vi "AttackerNormal.vi"(4 "AI Parameters":T1={"GotoKick"={"Dist do cone a frente"=150.0, "attacker farback"=1500.0, "Perto"=300.0, "min dist to kick"=150.0, "kick eps"=0.05, "Time to transition"=0.0}, "Attacker"={"CC chute"=0.09, "CC passe"=0.045, "Kick Force"=100.0, "D ball-robot Kick"=200.0, "D ball-robot Pass"=0.3}, "Defender"={"D max"=1700.0, "Vel p/ robô av"=1000.0, "Kick Force"=100.0, "D atk-def"=0.0, "D farback"=0.0}, "Timeout"={"Field/v in x"=6.0, "Dist Robots"=300, "Dist up in y"=300}, "Pose Striker"={"dist"=200.0, "Numeric"=-4.0, "dist 2"=200.0}, "Dist Stop"=300.0, "Distance when ball out"=200, "D central gap "=150.0, "T pass"=0.0, "Force ++"=0.0, "range kick"=0.0, "Chute alto"=TRUE, "Marcador novo"=TRUE} {"D central gap" format="%#_13g"; "Dist Stop" format="%#_13g"; "Pose Striker"."Numeric" format="%#_13g"; "Defender"."Kick Force" format="%#_13g"; "Defender"."Vel p/ robô av" format="%#_13g"; "Attacker"."D ball-robot Kick" format="%#_13g"; "Attacker"."Kick Force" format="%#_13g"; "Attacker"."CC passe" format="%#_13g"; "Attacker"."CC chute" format="%#_13g"; "GotoKick"."kick eps" format="%#_13g"; "GotoKick"."min dist to kick" format="%#_13g"; "GotoKick"."Perto" format="%#_13g"; "GotoKick"."attacker farback" format="%#_13g"; "GotoKick"."Dist do cone a frente" format="%#_13g"}, 5 "Penalty":bool, 7 "IA State Input 2":T3, 8 "atacando contra?":bool=TRUE, 9 "balls":T6[](array[typedef])=[{"x"=-974.5169677734375, "y"=-3444.3310546875, "timestamp"=timestamp(2082759045.994995 s since 1904-01-01), "Vel_x"=0.0, "Vel_y"=0.0, "Pos Bola Est"=[]}], 10 "Field Size in":T7={"line_width"=10, "field_length"=9000, "field_width"=6000, "boundary_width"=250, "referee_width"=425, "goal_width"=700, "goal_depth"=180, "goal_wall_width"=20, "center_circle_radius"=500, "defense_radius"=500, "defense_stretch"=350, "free_kick_from_defense_dist"=700, "penalty_spot_from_field_line_dist"=450, "penalty_line_from_spot_dist"=350}, 11 "Robot in":T4={"id"=5, "function"=enum."Attacker", "x"=-983.1382446289062, "y"=-3000.010498046875, "orientation"=-1.5516623258590698, "v_tangent"=0.0, "v_normal"=0.0, "v_ang"=0.0, "kick_x"=0.0, "kick_z"=0.0, "dribble"=FALSE, "Timestamp"=timestamp(2082759045.994995 s since 1904-01-01), "dest_x"=0.0, "dest_y"=0.0, "dest_orientation"=0.0, "estimatives"={"est_v_tangent"=0.0, "est_v_normal"=0.0, "est_vx"=0.0, "est_vy"=0.0, "Pos Robot Est"=[]}, "dest_x_kick"=0.0, "dest_y_kick"=0.0, "Gap Coord"=[], "States"=enum."GoToTangent", "Path "=[], "Path  Smooth"=[]}) -> (1 "Next State":T2=enum."GoToTangent", 2 "Robot out":T4={"id"=5, "function"=enum."Attacker", "x"=-983.1382446289062, "y"=-3000.010498046875, "orientation"=-1.5516623258590698, "v_tangent"=0.0001540345015520423, "v_normal"=0.008599927144915481, "v_ang"=0.002668461263266586, "kick_x"=0.0, "kick_z"=0.0, "dribble"=FALSE, "Timestamp"=timestamp(2082759045.994995 s since 1904-01-01), "dest_x"=0.0, "dest_y"=0.0, "dest_orientation"=0.0, "estimatives"={"est_v_tangent"=0.0, "est_v_normal"=0.0, "est_vx"=0.0, "est_vy"=0.0, "Pos Robot Est"=[]}, "dest_x_kick"=0.0, "dest_y_kick"=0.0, "Gap Coord"=[], "States"=enum."GoToTangent", "Path "=[], "Path  Smooth"=[]}, 3 "kick \nerror":dbl, 6 "Current States":T2=enum."GoToTangent")   [LabVIEW 2016]
uses:
  Core/AI Robot.ctl
  Functions Enum.ctl
  AttackerStates.ctl
  Core/Field Size.ctl
  Core/AI Ball.ctl
  Core/AI Input.ctl
  Core/AI Judge.ctl
  Command Enum.ctl
  Util/Events/Events.ctl
  AI Parameters.ctl
  <vilib>/Analysis/coordinate.llb/2D Cartesian Coordinate Rotation (Scalar).vi
  <vilib>/Analysis/NI_AALPro.lvlib
panel:
  in  "Cone de chute":dbl=0.9 format="%#_13g"
  out "Boolean":bool
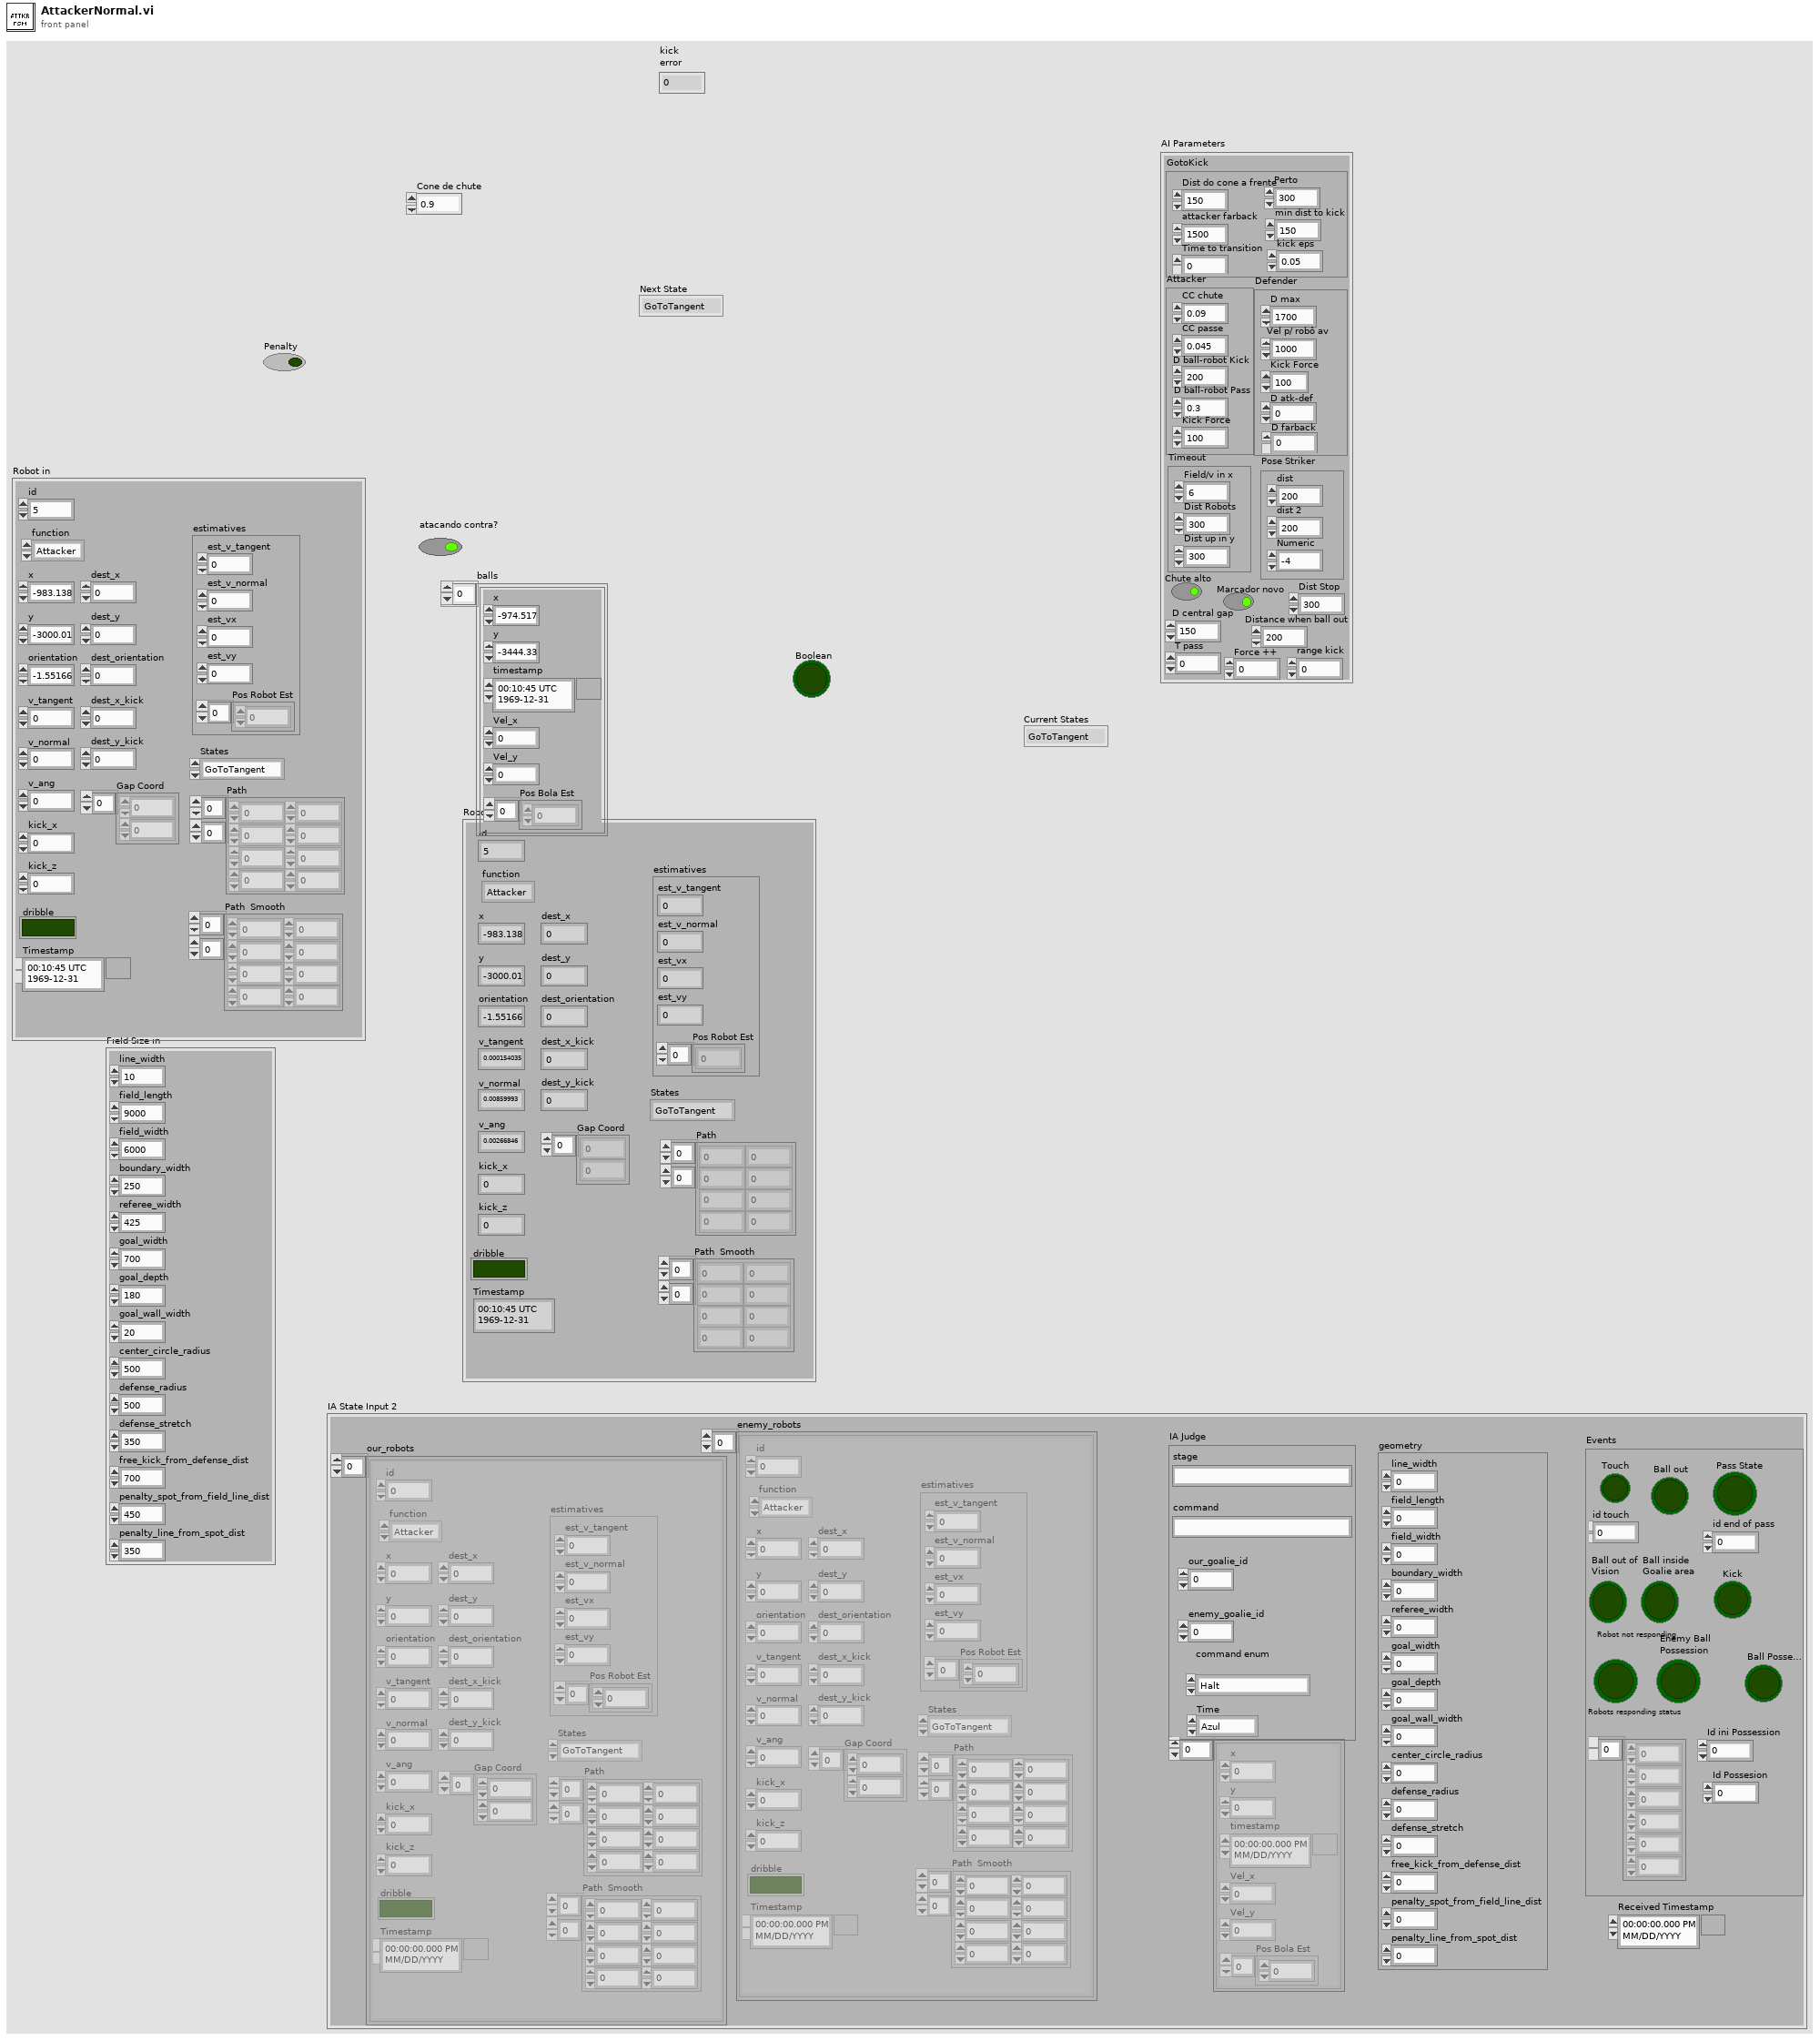
[diagram p1: front panel]
types:
  T1 = typedef "AI Parameters.ctl" = cluster{"GotoKick":cluster{"Dist do cone a frente":dbl, "attacker farback":dbl, "Perto":dbl, "min dist to kick":dbl, "kick eps":dbl, "Time to transition":dbl}, "Attacker":cluster{"CC chute":dbl, "CC passe":dbl, "Kick Force":dbl, "D ball-robot Kick":dbl, "D ball-robot Pass":dbl}, "Defender":cluster{"D max":dbl, "Vel p/ robô av":dbl, "Kick Force":dbl, "D atk-def":dbl, "D farback":dbl}, "Timeout":cluster{"Field/v in x":dbl, "Dist Robots":u32, "Dist up in y":u32}, "Pose Striker":cluster{"dist":dbl, "Numeric":dbl, "dist 2":dbl}, "Dist Stop":dbl, "Distance when ball out":i32, "D central gap ":dbl, "T pass":dbl, "Force ++":dbl, "range kick":dbl, "Chute alto":bool, "Marcador novo":bool}
  T2 = typedef "AttackerStates.ctl" = enum16{"Pass", "GoToTangent", "BallGetting", "GoToKick", ""}
  T3 = typedef "AI Input.ctl" = cluster{"our_robots":T4[], "enemy_robots":T4[], "balls":T6[], "geometry":T7, "IA Judge":T8, "Received Timestamp":timestamp, "Events":T10}
  T4 = typedef "AI Robot.ctl" = cluster{"id":u32, "function":T5, "x":dbl, "y":dbl, "orientation":dbl, "v_tangent":dbl, "v_normal":dbl, "v_ang":dbl, "kick_x":dbl, "kick_z":dbl, "dribble":bool, "Timestamp":timestamp, "dest_x":dbl, "dest_y":dbl, "dest_orientation":dbl, "estimatives":cluster{"est_v_tangent":dbl, "est_v_normal":dbl, "est_vx":dbl, "est_vy":dbl, "Pos Robot Est":dbl[]}, "dest_x_kick":dbl, "dest_y_kick":dbl, "Gap Coord":dbl[], "States":T2, "Path ":dbl[][], "Path  Smooth":dbl[][]}
  T5 = typedef "Functions Enum.ctl" = enum16{"Attacker", "Goalie", "Defender", "Striker", "Goto 0", "Dummy", "Kicker", "ZigZag"}
  T6 = typedef "AI Ball.ctl" = cluster{"x":dbl, "y":dbl, "timestamp":timestamp, "Vel_x":dbl, "Vel_y":dbl, "Pos Bola Est":dbl[]}
  T7 = typedef "Field Size.ctl" = cluster{"line_width":u32, "field_length":u32, "field_width":u32, "boundary_width":u32, "referee_width":u32, "goal_width":u32, "goal_depth":u32, "goal_wall_width":u32, "center_circle_radius":u32, "defense_radius":u32, "defense_stretch":u32, "free_kick_from_defense_dist":u32, "penalty_spot_from_field_line_dist":u32, "penalty_line_from_spot_dist":u32}
  T8 = typedef "AI Judge.ctl" = cluster{"stage":string, "command":string, "our_goalie_id":dbl, "enemy_goalie_id":dbl, "command enum":T9, "Time":enum16{"Azul", "Amarelo"}}
  T9 = typedef "Command Enum.ctl" = enum16{"Halt", "Stop", "Force Start", "PKA Normal Start", "Prepare Kickoff Ally", "PKE Normal Start", "Prepare Kickoff Enemy", "Prepare Penalty Ally", "PPA Normal Start", "Prepare Penalty Enemy", "PPE Normal Start", "Direct Free Enemy", "Direct Free Ally", "Indirect Free Enemy", "Indirect Free Ally", "Timeout Enemy", "Timeout Ally", "Goal Enemy", "Goal Ally", "Ball Placement Enemy", "Ball Placement Ally", "Normal Half Time", "Extra Time Break", "Extra Half Time", "None", "Post Game"}
  T10 = typedef "Events.ctl" = cluster{"Touch":bool, "Ball out":bool, "id touch":dbl, "Ball out of \nVision":bool, "Ball inside \nGoalie area":bool, "Robot not responding":bool, "Robots responding status":dbl[], "Enemy Ball \nPossession":bool, "Pass State":bool, "id end of pass":dbl, "Kick":bool, "Id ini Possession":dbl, "Ball Possesion":bool, "Id Possesion":dbl}
  T11 = cluster{"CC chute":dbl, "CC passe":dbl, "Kick Force":dbl, "D ball-robot Kick":dbl, "D ball-robot Pass":dbl}
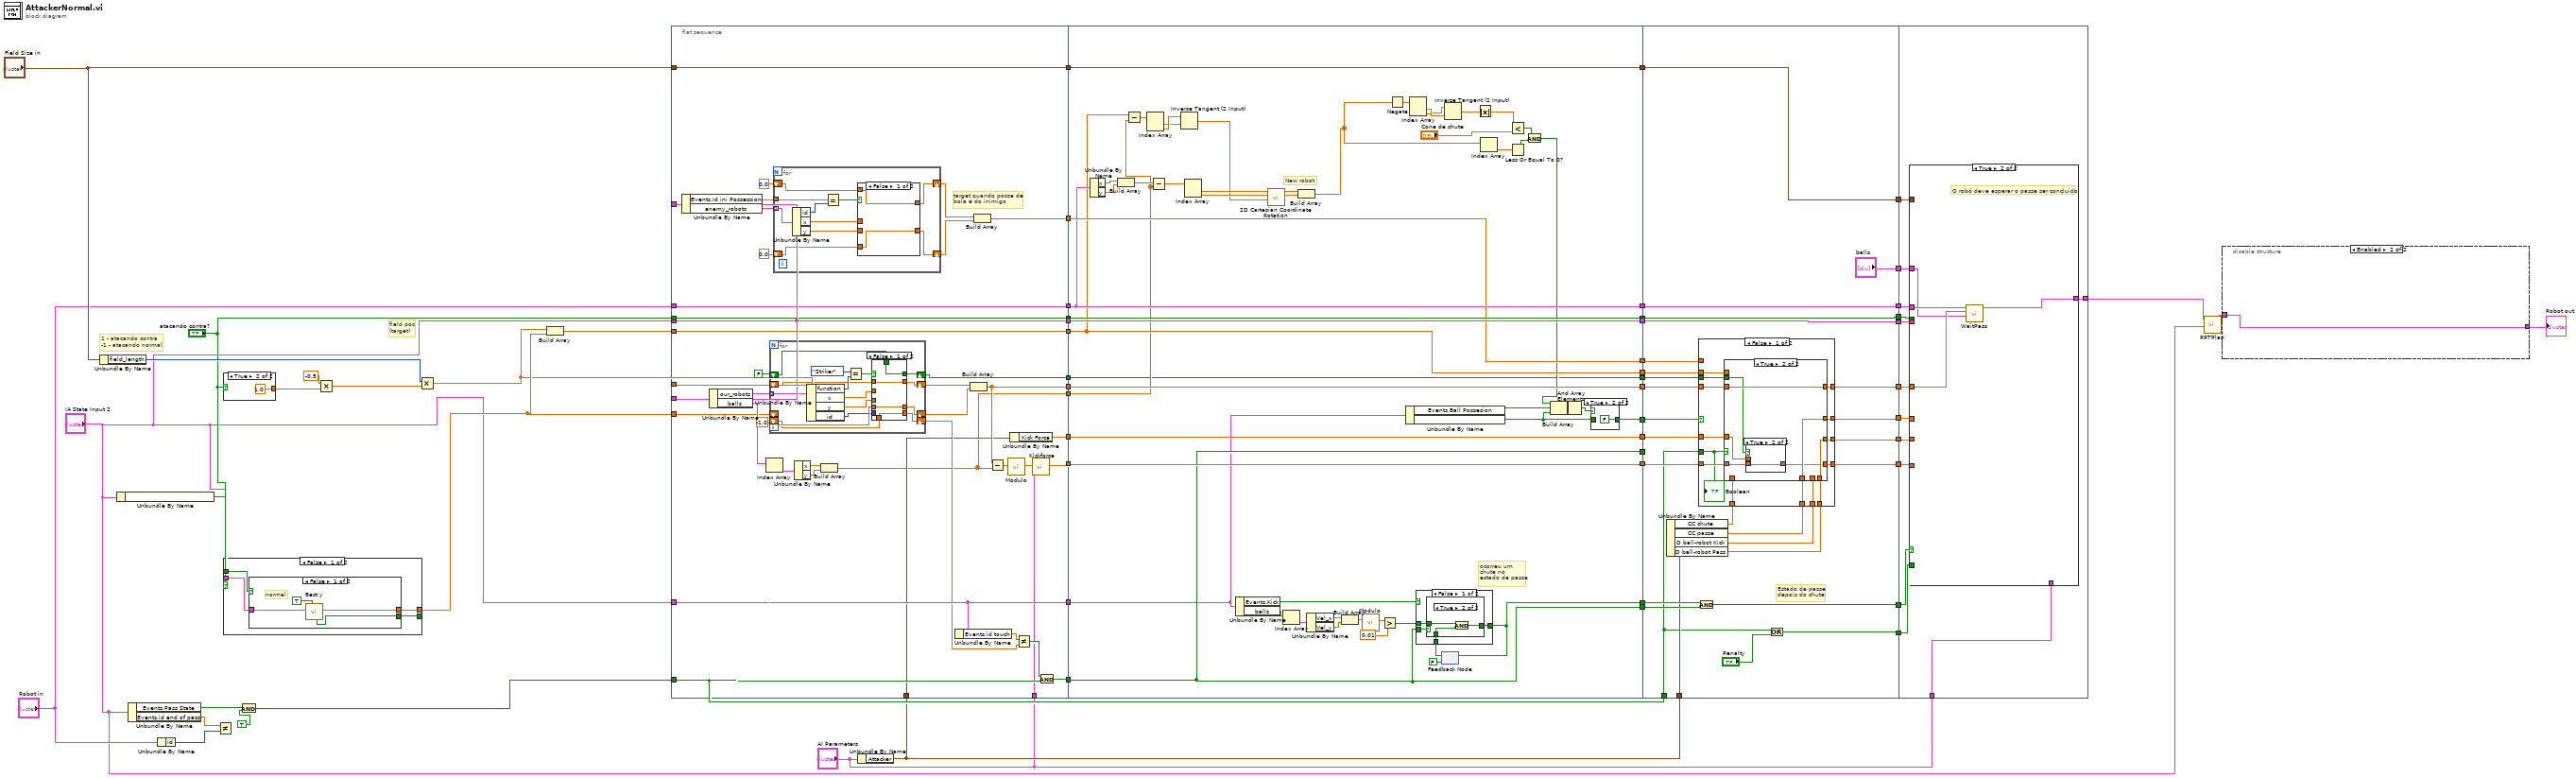
[diagram p0: block diagram]
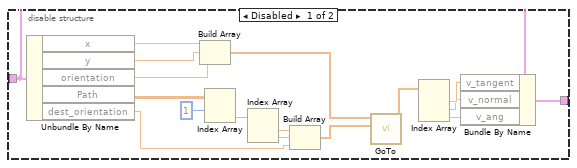
[diagram p2: hidden frame]
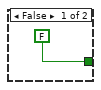
[diagram p6: hidden frame]
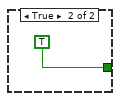
[diagram p7: hidden frame]
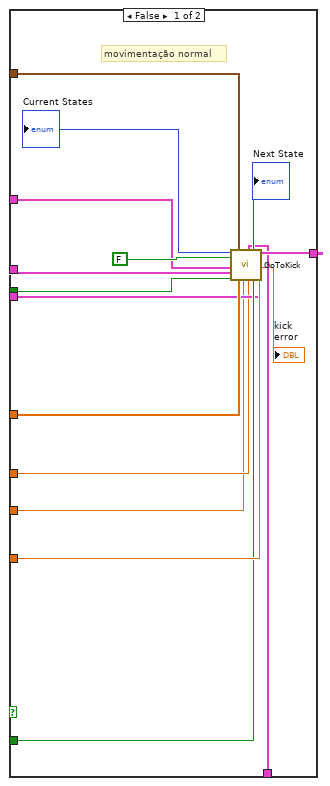
[diagram p11: hidden frame]
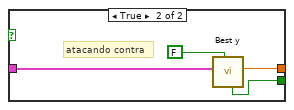
[diagram p12: hidden frame]
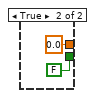
[diagram p13: hidden frame]
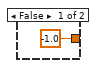
[diagram p14: hidden frame]
diagram:
  # "1 - atacando contra\n-1 - atacando normal"
  # "field pos\n(target)"
  n1 = Unbundle By Name("Field Size in") -> ("field_length"=w60:u32)
  n2 = Unbundle By Name("IA State Input 2") -> ("Events.Ball inside \nGoalie area"=w56:bool)
  n3 = Unbundle By Name("IA State Input 2") -> ("Events.Pass State"=w50:bool, "Events.id end of pass"=w52:dbl)
  n4 = Unbundle By Name("Robot in") -> ("id"=w51:u32)
  n5 = Not Equal?(x=w52, y=w51) -> ()  [unwired: 1 out]
  n6 = case shown="True" "atacando contra?" {
    tunnel: [-1.0 ("attck contra? 2") 1.0] -> w57
    frame False {
    }
    frame True {
    }
  }
  n7 = case shown="False" w56 {
    tunnel: "atacando contra?" -> [w66 _]
    tunnel: [w65 0.0] -> w28
    tunnel: "IA State Input 2" -> [w64 _]
    tunnel: [w63 FALSE ("Eclipse")] -> _
    frame False {
      n8 = case shown="False" w66 {
        tunnel: [w69 w73] -> w65
        tunnel: w64 -> [w67 w72]
        tunnel: [w68 w71] -> w63
        frame False {
          # "normal"
          n9 = call "Best y.vi"("inimigos"=TRUE, "IA State"=w67) -> ("Best y"=w69:dbl, "Eclipse"=w68:bool)  [unwired: 6 in, 2 out]
        }
        frame True {
          # "atacando contra"
          n10 = call "Best y.vi"("inimigos"=FALSE, "IA State"=w72) -> ("Best y"=w73:dbl, "Eclipse"=w71:bool)  [unwired: 6 in, 2 out]
        }
      }
    }
    frame True {
    }
  }
  n11 = And(x=w50, y=TRUE) -> (x .and. y?=w12:bool)
  n12 = Multiply(x=-0.5, y=w57) -> (x*y=w58:dbl)
  n13 = Multiply(x=w60, y=w58) -> (x*y=w27:dbl)
  n14 = Build Array(w27, w28) -> (w49:dbl[])
  n15 = flat-sequence {
    tunnel: "IA State Input 2" -> [w96]
    tunnel: w12 -> [w92]
    tunnel: w27 -> [w98]
    tunnel: w49 -> [w112]
    tunnel: "IA State Input 2" -> [w113]
    tunnel: "Robot in" -> [w114]
    tunnel: "Field Size in" -> [w115]
    tunnel: "atacando contra?" -> [w116]
    tunnel: [w116] -> w37
    tunnel: [w115] -> w36
    tunnel: [w114] -> w35
    tunnel: [w113] -> w34
    tunnel: [w99] -> w33
    tunnel: [w112] -> w32
    tunnel: [w100] -> w31
    tunnel: [w91] -> w30
    tunnel: [w96] -> w29
    tunnel: w28 -> [w102]
    tunnel: "IA State Input 2" -> [w101]
    tunnel: [w81] -> w26
    tunnel: "IA State Input 2" -> [w90]
    tunnel: [w85] -> w22
    tunnel: w10 -> [w82]
    tunnel: [w80] -> w8
    tunnel: [w78] -> w6
    tunnel: "AI Parameters" -> [w77]
    tunnel: [w206] -> w48
    tunnel: [w205] -> w47
    tunnel: [w179] -> w46
    tunnel: [w204] -> w45
    tunnel: [w197] -> w44
    tunnel: [w203] -> w43
    tunnel: [w202] -> w42
    tunnel: [w172] -> w41
    tunnel: [w201] -> w40
    tunnel: [w196] -> w39
    tunnel: [w196] -> w38
    tunnel: w37 -> [w206]
    tunnel: w36 -> [w205]
    tunnel: w35 -> [w179]
    tunnel: w34 -> [w204]
    tunnel: w33 -> [w202]
    tunnel: w32 -> [w172]
    tunnel: w31 -> [w201]
    tunnel: w30 -> [w196]
    tunnel: w29 -> [w195]
    tunnel: w26 -> [w203]
    tunnel: [w164] -> w24
    tunnel: [w194] -> w23
    tunnel: w22 -> [w194]
    tunnel: w8 -> [w171]
    tunnel: [w154] -> w7
    tunnel: w6 -> [w154]
    tunnel: w48 -> [w234]
    tunnel: w47 -> [w237]
    tunnel: w46 -> [w236]
    tunnel: w45 -> [w235]
    tunnel: w44 -> [w244]
    tunnel: w43 -> [w243]
    tunnel: w42 -> [w242]
    tunnel: w41 -> [w241]
    tunnel: w40 -> [w240]
    tunnel: w39 -> [w229]
    tunnel: w38 -> [_]
    tunnel: w24 -> [w239]
    tunnel: w23 -> [w238]
    tunnel: [w237] -> w21
    tunnel: [w236] -> w20
    tunnel: [w235] -> w19
    tunnel: [w234] -> w18
    tunnel: [w233] -> w17
    tunnel: [w232] -> w16
    tunnel: [w231] -> w15
    tunnel: [w230] -> w14
    tunnel: [w219] -> w13
    tunnel: w12 -> [w220]
    tunnel: ["balls"] -> w11
    tunnel: w10 -> [w227]
    tunnel: [w223] -> w9
    tunnel: w7 -> [w221]
    tunnel: w21 -> [w288]
    tunnel: w20 -> [w287]
    tunnel: w19 -> [w286]
    tunnel: w18 -> [w285]
    tunnel: w17 -> [w284]
    tunnel: w16 -> [w283]
    tunnel: w15 -> [w282]
    tunnel: w14 -> [w281]
    tunnel: w13 -> [w280]
    tunnel: [w279] -> w3
    tunnel: w11 -> [w278]
    tunnel: "AI Parameters" -> [w277]
    tunnel: w9 -> [w276]
    frame #0 {
      # "target quando posse de\nbola é do inimigo"
      n16 = Unbundle By Name(w90) -> ("Events.Id ini Possession"=w88:dbl, "enemy_robots"=w89:T4[])
      n17 = Unbundle By Name(w101) -> ("our_robots"=w103:T4[], "balls"=w106:T6[])
      n18 = Index Array(array=w106) -> (element=w107:T6)  [unwired: 1 in]
      n19 = for {
        tunnel: w103 -> [w145] mode=indexing
        shift-right: [w140] -> w104
        shift-left: w98 -> [w139]
        shift-right: [w137] -> w105
        shift-left: w102 -> [w136]
        shift-right: [w134] -> w94
        shift-left: -1.0 -> [w133]
        shift-right: [w131] -> w78
        shift-left: FALSE -> [w132]
        n20 = Unbundle By Name(w145) -> ("function"=w144:T5, "x"=w141:dbl, "y"=w138:dbl, "id"=w135:u32)
        n21 = Equal?(x=Functions_Enum."Striker", y=w144) -> (x = y?=w142:bool)
        n22 = case shown="False" w142 {
          selector: w142 -> [_ w150]
          tunnel: [w149 w153] -> w140
          tunnel: w141 -> [_ w153]
          tunnel: w139 -> [w149 _]
          tunnel: w138 -> [_ w152]
          tunnel: [w148 w152] -> w137
          tunnel: w136 -> [w148 _]
          tunnel: w135 -> [_ w151]
          tunnel: [w147 w151] -> w134
          tunnel: w133 -> [w147 _]
          tunnel: w132 -> [w146 _]
          tunnel: [w146 w150] -> w131
          frame False {
          }
          frame True {
          }
        }
      }
      n23 = for {
        tunnel: w89 -> [w126] mode=indexing
        tunnel: w88 -> [w124]
        shift-right: [w120] -> w87
        shift-left: 0.0 ("x") -> [w118]
        shift-right: [w119] -> w86
        shift-left: 0.0 ("y") -> [w117]
        n24 = Unbundle By Name(w126) -> ("id"=w125:u32, "x"=w122:dbl, "y"=w121:dbl)
        n25 = Equal?(x=w124, y=w125) -> (x = y?=w123:bool)
        n26 = case shown="False" w123 {
          tunnel: w122 -> [_ w130]
          tunnel: w121 -> [_ w129]
          tunnel: [w128 w130] -> w120
          tunnel: [w127 w129] -> w119
          tunnel: w118 -> [w128 _]
          tunnel: w117 -> [w127 _]
          frame False {
          }
          frame True {
          }
        }
      }
      n27 = Unbundle By Name(w107) -> ("x"=w108:dbl, "y"=w109:dbl)
      n28 = Build Array(w108, w109) -> (w80:dbl[])
      n29 = Unbundle By Name(w96) -> ("Events.id touch"=w95:dbl)
      n30 = Build Array(w104, w105) -> (w100:dbl[])
      n31 = Build Array(w87, w86) -> (w85:dbl[])
      n32 = Subtract(x=w100, y=w80) -> (x-y=w110:dbl[])
      n33 = call "Modulo.vi"("2D vector"=w110) -> ("Modulo"=w111:dbl)  [unwired: 10 in]
      n34 = Unbundle By Name(w82) -> ("Kick Force"=w81:dbl)
      n35 = Not Equal?(x=w95, y=w94) -> (x != y?=w93:bool)
      n36 = call "Kickforce.vi"("AI Parameters"=w77, "Distância ao\nalvo do chute"=w111) -> ("Força do chute"=w99:dbl)  [unwired: 8 in, 1 out]
      n37 = And(x=w93, y=w92) -> (x .and. y?=w91:bool)
    }
    frame #1 {
      # "New robot"
      # "ocorreu um \nchute no\nestado de passe"
      n38 = Unbundle By Name(w179) -> ("x"=w178:dbl, "y"=w177:dbl)
      n39 = Build Array(w178, w177) -> (w176:dbl[])
      n40 = Subtract(x=w172, y=w171) -> (x-y=w173:dbl[])
      n41 = Index Array(array=w173) -> (element #1=w174:dbl, element #2=w175:dbl)  [unwired: 2 in]
      n42 = Subtract(x=w176, y=w171) -> (x-y=w182:dbl[])
      n43 = Inverse Tangent (2 Input)(1:w174, 2:w175) -> (0:w170:dbl)
      n44 = Index Array(array=w182) -> (element #1=w184:dbl, element #2=w183:dbl)  [unwired: 2 in]
      n45 = Unbundle By Name(w195) -> ("Events.Kick"=w198:bool, "balls"=w162:T6[])
      n46 = call-poly <vilib>:"2D Cartesian Coordinate Rotation.vi"("theta"=w170, "y"=w183, "x"=w184) -> ("y out"=w180:dbl, "x out"=w181:dbl)  [unwired: 6 in, 1 out]
      n47 = Index Array(array=w162) -> (element=w161:T6)  [unwired: 1 in]
      n48 = Build Array(w181, w180) -> (w169:dbl[])
      n49 = Unbundle By Name(w161) -> ("Vel_x"=w160:dbl, "Vel_y"=w159:dbl)
      n50 = Build Array(w160, w159) -> (w158:dbl[])
      n51 = call "Modulo.vi"("2D vector"=w158) -> ("Modulo"=w157:dbl)  [unwired: 10 in]
      n52 = Greater?(x=w157, y=0.01) -> (0:w155:bool)
      n53 = Negate(x=w169) -> (-x=w193:dbl[])
      n54 = Unbundle By Name(w195) -> ("Events.Ball Possesion"=w167:bool, "Events.Enemy Ball \nPossession"=w163:bool)
      n55 = Index Array(array=w193) -> (element #1=w192:dbl, element #2=w191:dbl)  [unwired: 2 in]
      n56 = feedback #1(FALSE) -> (w199:bool)
      n57 = case shown="False" w198 {
        tunnel: [w211 TRUE] -> w197
        tunnel: w199 -> [w210 _]
        tunnel: w196 -> [w212 _]
        tunnel: w155 -> [w209 _]
        frame False {
          n58 = case shown="True" w212 {
            tunnel: [FALSE w216] -> w211
            tunnel: w210 -> [_ w215]
            tunnel: w209 -> [_ w214]
            frame False {
            }
            frame True {
              n59 = And(x=w214, y=w215) -> (x .and. y?=w216:bool)
            }
          }
        }
        frame True {
        }
      }
      n60 = feedback-in #1(w197) -> ()
      n61 = Inverse Tangent (2 Input)(1:w192, 2:w191) -> (0:w190:dbl)
      n62 = Absolute Value(x=w190) -> (abs(x)=w185:dbl)
      n63 = Index Array(array=w169) -> (element=w188:dbl)  [unwired: 1 in]
      n64 = Less?(x=w185, y="Cone de chute") -> (x < y?=w187:bool)
      n65 = Less Or Equal To 0?(x=w188) -> (x <= 0?=w186:bool)
      n66 = And(x=w187, y=w186) -> (x .and. y?=w166:bool)
      n67 = Build Array(w166, w167, w163) -> (w168:bool[])
      n68 = And Array Elements(Boolean array=w168) -> (logical AND=w165:bool)
      n69 = case shown="True" w165 {
        tunnel: [w207 FALSE] -> w164
        tunnel: w163 -> [w207 _]
        frame False {
        }
        frame True {
        }
      }
    }
    frame #2 {
      # "Estado de passe\ndepois do chute"
      n70 = Unbundle By Name(w227) -> ("CC chute"=w226:dbl, "CC passe"=w225:dbl, "D ball-robot Kick"=w224:dbl, "D ball-robot Pass"=w222:dbl)
      n71 = And(x=w244, y=w229) -> (x .and. y?=w230:bool)
      n72 = case shown="False" w239 {
        tunnel: w243 -> [w258 w275]
        tunnel: w242 -> [w257 _]
        tunnel: w241 -> [w256 _]
        tunnel: w240 -> [w255 _]
        tunnel: [w254 w274] -> w233
        tunnel: [w253 w275] -> w231
        tunnel: w220 -> [w252 _]
        tunnel: w238 -> [_ w274]
        tunnel: [w251 w273] -> w232
        tunnel: w226 -> [w250 w273]
        tunnel: w225 -> [w249 _]
        tunnel: w224 -> [w248 w272]
        tunnel: [w247 w272] -> w223
        tunnel: w222 -> [w246 _]
        tunnel: w221 -> [w245 _]
        frame False {
          n73 = case shown="True" w252 {
            tunnel: w258 -> [w261 w263]
            tunnel: w257 -> [_ w265]
            tunnel: w256 -> [w262 _]
            tunnel: w255 -> [_ w269]
            tunnel: [w262 w269] -> w254
            tunnel: [w261 w264] -> w253
            tunnel: [w260 w268] -> w251
            tunnel: w250 -> [w260 _]
            tunnel: w249 -> [_ w268]
            tunnel: [w259 w267] -> w247
            tunnel: w248 -> [w259 _]
            tunnel: w246 -> [_ w267]
            tunnel: w245 -> [_ w266]
            frame False {
            }
            frame True {
              n74 = case shown="True" w266 {
                tunnel: [w270 w271] -> w264
                tunnel: w265 -> [_ w271]
                tunnel: w263 -> [w270 _]
                frame False {
                }
                frame True {
                }
              }
            }
          }
          "Boolean" <- w252
        }
        frame True {
        }
      }
      n75 = Or(x=w220, y="Penalty") -> (x .or. y?=w219:bool)
    }
    frame #3 {
      n76 = case shown="True" w281 {
        tunnel: w285 -> [w302 _]
        tunnel: w288 -> [w301 _]
        tunnel: w287 -> [w300 w307]
        tunnel: w284 -> [w299 w306]
        tunnel: w282 -> [w298 _]
        tunnel: w280 -> [w297 _]
        tunnel: w286 -> [w296 _]
        tunnel: [w295 w308] -> w279
        tunnel: w283 -> [w293 _]
        tunnel: w278 -> [w292 w305]
        tunnel: w277 -> [w291 _]
        tunnel: w276 -> [w289 _]
        frame False {
          # "movimentação normal"
          n77 = call "GoToKick.vi"("goleiro?"=FALSE, "balls"=w292, "Robot in in"=w300, "atacando contra?"=w302, "Field Size in"=w301, "Target"=w299, "D ball - robot"=w289, "AI Parameters"=w291, "Cone de chute"=w293, "Passe"=w297, "Kick Force"=w298, "IA State Input in"=w296) -> ("Current States"=→"Current States":T2, "Next State"=→"Next State":T2, "Robot out"=w295:T4, "kick error"=→"kick \nerror":dbl)  [unwired: 4 in]
        }
        frame True {
          # "O robô deve esperar o passe ser concluido"
          n78 = call "WaitPass.vi"("balls"=w305, "Target"=w306, "Robot in"=w307) -> ("Robot out"=w308:T4)  [unwired: 8 in]
        }
      }
    }
  }
  n79 = Unbundle By Name("AI Parameters") -> ("Attacker"=w10:T11)
  n80 = call "RRTPlan.vi"("IA State"="IA State Input 2", "Robot"=w3) -> ("Robot Out"=w1:T4)  [unwired: 9 in]
  n81 = disable-structure shown="Enabled" {
    disable-tunnel: [w325 w326] -> w2
    disable-tunnel: w1 -> [w315 w326]
    frame Disabled {
      n82 = Unbundle By Name(w315) -> ("x"=w319:dbl, "y"=w318:dbl, "orientation"=w317:dbl, "Path"=w324:dbl[][], "dest_orientation"=w310:dbl)
      n83 = Build Array(w319, w318, w317) -> (w316:dbl[])
      n84 = Index Array(array=w324, index (row)=1) -> (element=w322:dbl[])  [unwired: 1 in]
      n85 = Index Array(array=w322) -> (element #1=w321:dbl, element #2=w320:dbl)  [unwired: 2 in]
      n86 = Build Array(w321, w320, w310) -> (w309:dbl[])
      n87 = call "GoTo.vi"("Target"=w309, "Position"=w316) -> ("Output\nVelocity"=w314:dbl[])  [unwired: 8 in, 1 out]
      n88 = Index Array(array=w314) -> (element #1=w313:dbl, element #2=w312:dbl, element #3=w311:dbl)  [unwired: 3 in]
      n89 = Bundle By Name(cluster=w315, "v_tangent"=w313, "v_normal"=w312, "v_ang"=w311) -> (w325:T4)
    }
    frame Enabled {
    }
  }
  "Robot out" <- w2
